vi "Update Result.vi"(7 "Result Table In":string[][](table), 8 "error in (no error)":errorcluster, 9 "Mic 2 Result":T1, 10 "Mic 1 Result":T1, 11 "PSU":cluster{"Current (mA)":dbl, "Voltage (V)":dbl}) -> (0 "error out":errorcluster, 5 "Result Table Out":string[][](table))   [LabVIEW 2018]
panel:
  in  "Update Result":enum16{"PSU", "MIC 1", "MIC 2"}(ring)
  # "Update Test Data Result"
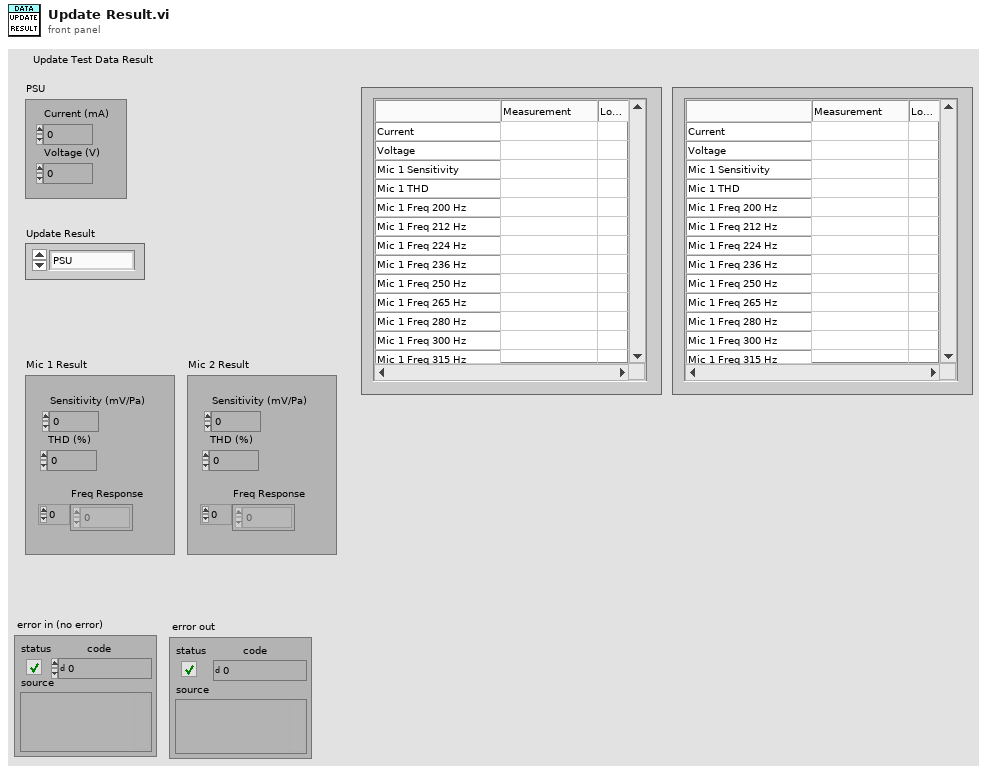
[diagram p1: front panel]
types:
  T1 = cluster{"Sensitivity (mV/Pa)":dbl, "THD (%)":dbl, "Freq Response":dbl[]}
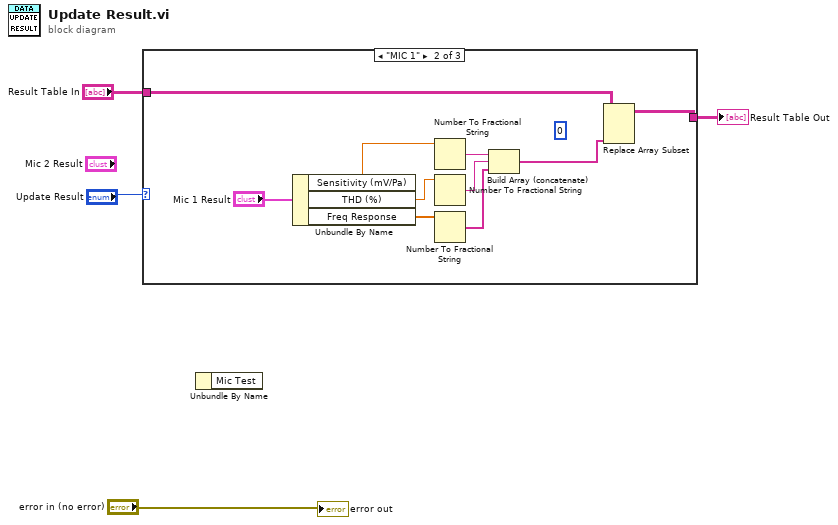
[diagram p0: block diagram]
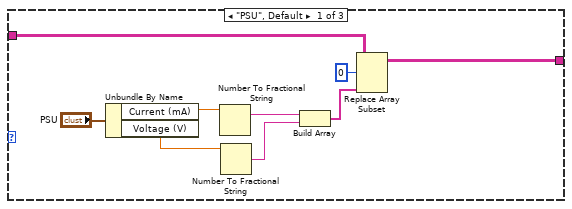
[diagram p2: hidden frame]
diagram:
  n1 = case shown="\"MIC 1\"" "Update Result" {
    tunnel: "Result Table In" -> [w8 w16 _]
    tunnel: [w5 w14 _] -> w1
    frame "PSU", Default {
      n2 = Unbundle By Name("PSU") -> ("Current (mA)"=w12:dbl, "Voltage (V)"=w11:dbl)
      n3 = Number To Fractional String(number=w12) -> (F-format string=w10:string)  [unwired: 3 in]
      n4 = Number To Fractional String(number=w11) -> (F-format string=w9:string)  [unwired: 3 in]
      n5 = Build Array(w10, w9) -> (w7:string[])
      n6 = Replace Array Subset(array=w8, new element=w7, index (row)=0) -> (w5:string[][])  [unwired: 1 in]
    }
    frame "MIC 1" {
      (unwired) 0 ("index (row)")
      n7 = Unbundle By Name("Mic 1 Result") -> ("Sensitivity (mV/Pa)"=w22:dbl, "THD (%)"=w21:dbl, "Freq Response"=w23:dbl[])
      n8 = Number To Fractional String(number=w22) -> (F-format string=w20:string)  [unwired: 3 in]
      n9 = Number To Fractional String(number=w21) -> (F-format string=w19:string)  [unwired: 3 in]
      n10 = Number To Fractional String(number=w23) -> (F-format string=w18:string[])  [unwired: 3 in]
      n11 = Build Array (concatenate)(w20, w19, w18) -> (w15:string[])
      n12 = Replace Array Subset(array=w16, new element=w15) -> (w14:string[][])  [unwired: 2 in]
    }
    frame "MIC 2" {
    }
  }
  "Result Table Out" <- w1
  n13 = Unbundle By Name() -> ()  [unwired: 1 in, 1 out]
  "error out" <- "error in (no error)"
